vi "Stop Core.vi"(10 "final error code":i32, 11 "Mediator in":refnum<class "Mediator.lvclass">) -> (3 "Mediator out":refnum<class "Mediator.lvclass">)   [LabVIEW 2017, in "Mediator.lvlib" / "Mediator.lvclass"]
doc: "(<B>Filename</B>: Actor Framework.lvlib:Actor.lvclass:Stop Core.vi)\n\nDefines what the actor does before it stops. Use the <B>final error code</B> input to determine whether the actor shut down in response to an error.\n\nBy default, this method does nothing. A descendant class may override it to define behavior, such as shutting down any processes the actor initiated in its override of the Actor Core method."
uses:
  Mediator.lvclass
  Mediator.lvclass/Mediator.ctl
  <vilib>/ActorFramework/Message Enqueuer/Message Enqueuer.lvclass/Message Enqueuer.ctl
  <vilib>/ActorFramework/Message Enqueuer/Enqueue.vi
  <vilib>/ActorFramework/Stop Msg/Stop Msg.lvclass
  C:/Program Files (x86)/National Instruments/LabVIEW 2017/vi.lib/ActorFramework/Message/Message.lvclass
  <vilib>/ActorFramework/Message Priority Queue/Priority Enqueue.vi
  IMediator/IMediator/IMediator.lvclass
  TopicLookupTable/TopicLookupTable.lvclass
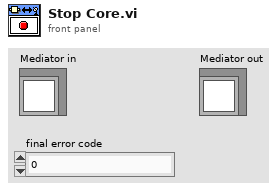
[diagram p1: front panel]
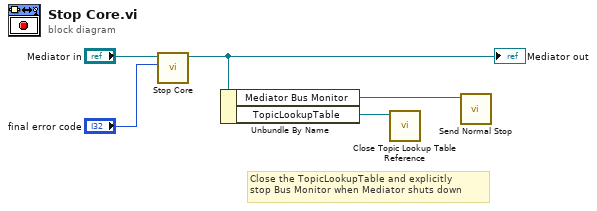
[diagram p0: block diagram]
diagram:
  # "Close the TopicLookupTable and explicitly\nstop Bus Monitor when Mediator shuts down"
  n1 = call-parent "Stop Core.vi"("final error code"="final error code", "Mediator In"="Mediator in") -> ("Mediator Out"=w3:refnum<class "Mediator.lvclass">)  [unwired: 9 in]
  "Mediator out" <- w3
  n2 = Unbundle By Name(w3) -> ("Mediator Bus Monitor"=w1:refnum<class "Message Enqueuer.lvclass">, "TopicLookupTable"=w2:refnum<data-value>)
  n3 = call "Close Topic Lookup Table Reference.vi"("TopicLookupTable"=w2) -> ()  [unwired: 10 in, 1 out]
  n4 = call <vilib>:"Send Normal Stop.vi"("Message Enqueuer"=w1) -> ()  [unwired: 10 in, 1 out]
